vi "ZLIB Compress Directory__ogtk.vi"(6 "password (none)":string, 7 "append (create new)":T1, 8 "error in (no error)":errorcluster, 9 "include subdirectories (F)":bool, 10 "archive name (root directory with .zip ending)":path, 11 "root directory (file dialog)":path) -> (0 "error out":errorcluster, 2 "archive name out":path, 3 "root directory out":path)   [LabVIEW 2011]
doc: "This function compresses an entire directory and eventually its subdirectories into a ZIP file. The root directory must be defined and if no root directory is passed to the function it will prompt the user for such a directory with the file dialog. If no archive name is specified this function will create a file with the same name and in the same location as the root directory, by removing any possible extension from the root directory name and appending the ending .zip to it.\n\nInclude subdirectories will control if this function recursively includes any subdirectories and its content from the root directory.\n\npassword, if not empty, will encrypt all the newly added files in the archive in such a way that they can only be extracted with the password later on."
uses:
  ZLIB Open ZIP Mode__ogtk.ctl
  file/file.llb/Valid Path - Traditional__ogtk.vi
  file/file.llb/Convert File Extension (Path)__ogtk.vi
  file/file.llb/Compare Two Paths - Scalar__ogtk.vi
  ZLIB Store File__ogtk.vi
panel:
  # "Please visit http://www.OpenG.org to learn about the\nOpen Source LabVIEW software movement.\n\nNOTICE -- YOU MUST LEAVE THIS NOTICE IN PLACE.  PER THE TERMS OF THE LICENSE BELOW, YOU MAY SUBLICENSE THIS SOFTWARE \nIN ANY WAY THAT DOES NOT CONFLICT WITH THIS LICENSE.\n\n### BSD License (http://www.opensource.org/licenses/bsd-license.php) Begin ###\n \nCopyright (C) 2002-2004 Rolf Kalbermatter rolf.kalbermatter@citeng.com\nCopyright (C) 2002 Jim Kring jim@jimkring.com\n\nAll rights reserved.\n\nRedistribution and use in source and binary forms, with or without modification, are permitted provided that the following conditions are met:\n\n    * Redistributions of source code must retain the above copyright notice, this list of conditions and the following disclaimer.\n    * Redistributions in binary form must reproduce the above copyright notice, this list of conditions and the following disclaimer in the \n       documentation and/or other materials provided with the distribution.\n    * Neither the name of SciWare, James Kring, Inc., nor the names of its contributors may be used to endorse or promote products derived \n       from this software without specific prior written permission.\n\nTHIS SOFTWARE IS PROVIDED BY THE COPYRIGHT HOLDERS AND CONTRIBUTORS \"AS IS\" AND ANY EXPRESS OR IMPLIED WARRANTIES, \nINCLUDING, BUT NOT LIMITED TO, THE IMPLIED WARRANTIES OF MERCHANTABILITY AND FITNESS FOR A PARTICULAR PURPOSE ARE \nDISCLAIMED. IN NO EVENT SHALL THE COPYRIGHT OWNER OR CONTRIBUTORS BE LIABLE FOR ANY DIRECT, INDIRECT, INCIDENTAL,\n SPECIAL, EXEMPLARY, OR CONSEQUENTIAL DAMAGES (INCLUDING, BUT NOT LIMITED TO, PROCUREMENT OF SUBSTITUTE GOODS OR \nSERVICES; LOSS OF USE, DATA, OR PROFITS; OR BUSINESS INTERRUPTION) HOWEVER CAUSED AND ON ANY THEORY OF LIABILITY, \nWHETHER IN CONTRACT, STRICT LIABILITY, OR TORT (INCLUDING NEGLIGENCE OR OTHERWISE) ARISING IN ANY WAY OUT OF THE USE \nOF THIS SOFTWARE, EVEN IF ADVISED OF THE POSSIBILITY OF SUCH DAMAGE.\n\n### BSD License End ###"
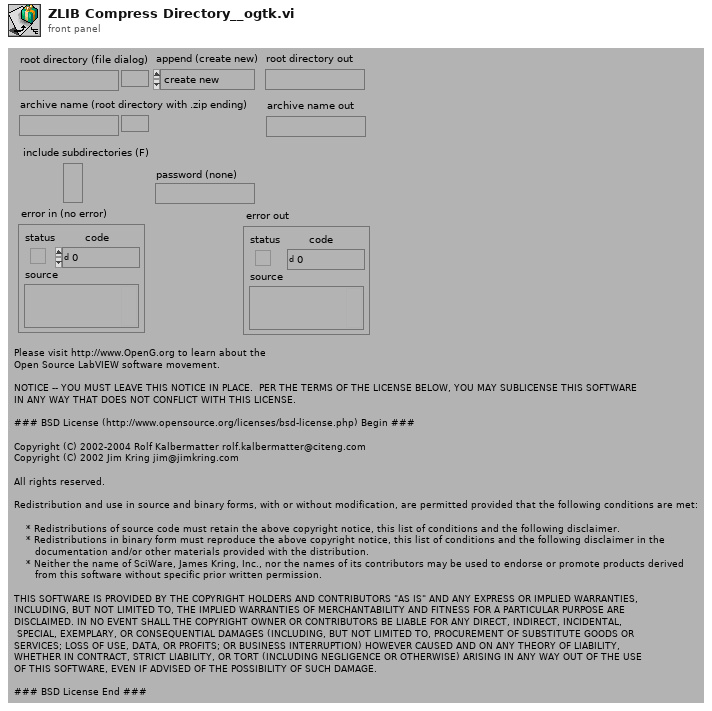
[diagram p1: front panel]
types:
  T1 = typedef "ZLIB Open ZIP Mode__ogtk.ctl" = enum16{"create new", "append to end", "append to archive"}
  T2 = enum32{"existing file", "new file", "new or existing file", "existing dir", "new dir", "new or existing dir", "existing file (use LLBs)", "new file (use LLBs)", "new or existing file (use LLBs)", "new or existing file or directory (use LLBs)", "existing dir (use LLBs)", "new dir (use LLBs)", "new or existing dir (use LLBs)", "existing file or dir", "new file or dir", "new or existing file or dir", "existing file or dir (use LLBs)", "new file or dir (use LLBs)"}
  T3 = typedef "ZLIB Zip Handle__ogtk.ctl" = refnum<k1>
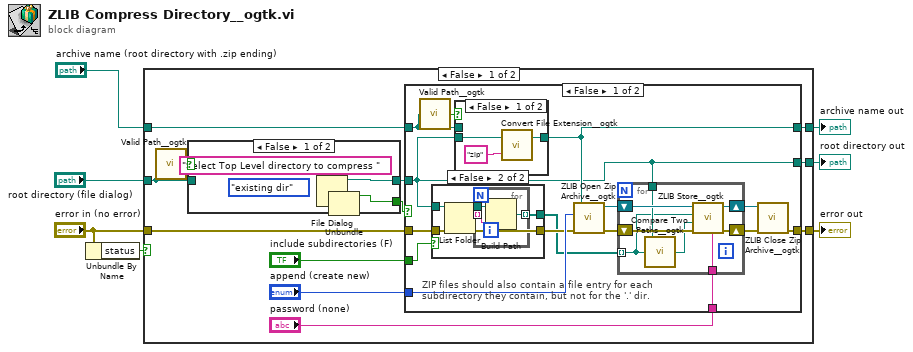
[diagram p0: block diagram]
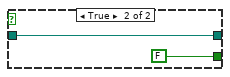
[diagram p2: hidden frame]
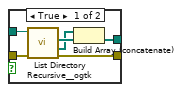
[diagram p3: hidden frame]
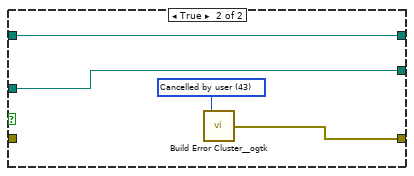
[diagram p5: hidden frame]
diagram:
  n1 = Unbundle By Name("error in (no error)") -> ("status"=w6:bool)
  n2 = case shown="False" w6 {
    tunnel: "root directory (file dialog)" -> [w16 w73]
    tunnel: "error in (no error)" -> [w13 w74]
    tunnel: [w14 w74] -> w4
    tunnel: [w12 w73] -> w3
    tunnel: [w11 w72] -> w2
    tunnel: "archive name (root directory with .zip ending)" -> [w10 w72]
    frame False {
      n3 = call-poly "Valid Path__ogtk.vi"("path"=w16) -> ("valid"=w17:bool)
      n4 = case shown="False" w17 {
        tunnel: [w22 w25] -> w19
        tunnel: [w21 FALSE ("cancelled")] -> w18
        tunnel: w16 -> [_ w25]
        frame False {
          (unwired) T2."existing dir" ("select mode (2)")
          n5 = File Dialog(7:"Select Top Level directory to compress " ("prompt")) -> (0:w20:errorcluster, 1:w21:bool, 3:w22:path)  [unwired: 6 in, 1 out]
          n6 = Unbundle(w20) -> ()  [unwired: 3 out]
        }
        frame True {
        }
      }
      n7 = case shown="False" w18 {
        tunnel: w19 -> [w31 w69]
        tunnel: w10 -> [w35 w68]
        tunnel: "include subdirectories (F)" -> [w28 _]
        tunnel: [w34 w71] -> w14
        tunnel: w13 -> [w30 _]
        tunnel: [w31 w69] -> w12
        tunnel: [w33 w68] -> w11
        tunnel: "append (create new)" -> [w32 _]
        tunnel: "password (none)" -> [w26 _]
        frame False {
          # "ZIP files should also contain a file entry for each\nsubdirectory they contain, but not for the '.' dir."
          n8 = call-poly "Valid Path__ogtk.vi"("path"=w35) -> ("valid"=w36:bool)
          n9 = case shown="False" w28 {
            tunnel: w31 -> [w46 w52]
            tunnel: [w42 w48] -> w27
            tunnel: w30 -> [w44 w51]
            tunnel: [w43 w47] -> w29
            frame True {
              n10 = call "List Directory Recursive__ogtk.vi"("error in (no error)"=w44, "Path"=w46) -> ("error out"=w43:errorcluster, "dir paths"=w41:path[], "file paths"=w45:path[])  [unwired: 6 in, 1 out]
              n11 = Build Array (concatenate)(w41, w45) -> (w42:path[])
            }
            frame False {
              n12 = List Folder(path=w52, error in=w51) -> (path out=w50:path, filenames=w49:string[], error out=w47:errorcluster)  [unwired: 2 in, 1 out]
              n13 = for {
                tunnel: w50 -> [w55]
                tunnel: w49 -> [w54] mode=indexing
                tunnel: [w53] -> w48 mode=indexing
                n14 = Build Path(base path=w55, name or relative path=w54) -> (appended path=w53:path)
              }
            }
          }
          n15 = case shown="False" w36 {
            tunnel: [w56 w59] -> w33
            tunnel: w31 -> [w57 _]
            tunnel: w35 -> [_ w59]
            frame False {
              n16 = call-poly "Convert File Extension__ogtk.vi"("new ending (none)"="zip" ("Format String"), "file name"=w57) -> ("new filename"=w56:path)  [unwired: 1 out]
            }
            frame True {
            }
          }
          n17 = call "ZLIB Open Zip Archive__ogtk.vi"("error in (no error)"=w29, "append (create new)"=w32, "archive name"=w33) -> ("error out"=w40:errorcluster, "zip Refnum"=w39:T3)  [unwired: 2 in, 1 out]
          n18 = for {
            shift-right: [w65] -> w38
            shift-left: w39 -> [w67]
            shift-right: [w64] -> w37
            shift-left: w40 -> [w66]
            tunnel: w27 -> [w62] mode=indexing
            tunnel: w31 -> [w63]
            tunnel: w26 -> [w60]
            n19 = call-poly "Compare Two Paths__ogtk.vi"("path2"=w62, "path1"=w63) -> ("relative path from 1 to 2"=w61:path)  [unwired: 1 in, 2 out]
            n20 = call-poly "ZLIB Store__ogtk.vi"("password (none)"=w60, "error in (no error)"=w66, "internal name (same as source name)"=w61, "source path"=w62, "zip Refnum"=w67) -> ("error out"=w64:errorcluster, "zip Refnum out"=w65:T3)  [unwired: 5 in]
          }
          n21 = call "ZLIB Close Zip Archive__ogtk.vi"("error in (no error)"=w37, "zip Refnum"=w38) -> ("error out"=w34:errorcluster)  [unwired: 4 in, 1 out]
        }
        frame True {
          w70 = 43 items=["No error", "Argument error", "Memory is full", "Out of zone", "End of file", "File already open", "Generic file I/O error", "File not found", "File permission error", "Disk is full", "Duplicate path", "Too many files open", "System feature not enabled", "Resource file not found", "Cannot add resource", "Resource not found", "Image not found", "Image memory error", "Pen does not exist", "Config type invalid", "Config token not found", "Config parse error", "Config memory error", "Bad external code format", "Bad external code offset", "External code not present", "Null window", "Destroy window error", "Null menu", "Print aborted", "Bad print record", "Print driver error", "Windows error during printing", "Memory error during printing", "Print dialog error", "Generic print error", "Invalid device refnum", "Device not found", "Device parameter error", "Device unit error", "Cannot open device", "Device call aborted", "Generic error", "Cancelled by user", "Object ID too low", "Object ID too high", "Object not in heap", "Unknown heap", "Unknown object (invalid DefProc)", "Unknown object (DefProc not in table)", "Message out of range", "Invalid (null) method", "Unknown message", "Manager call not supported", "Bad address", "Network operation in progress", "Network operation timed out", "Connection is busy", "Network attribute not supported", "Network error", "Address in use", "System out of memory", "Connection aborted", "Connection refused", "Not connected", "Already connected", "Connection closed", "Initialization error (interapplication manager)", "Bad occurrence", "Wait on unbound occurrence handler", "Occurrence queue overflow", "Datalog type conflict", "Unused", "Unrecognized type (interapplication manager)", "Memory corrupt", "Failed to make temporary DLL", "Old CIN version", "Drag socket not found", "Failed to load drop-object", "Failed to register OLE object", "Failed to release OLE object", "Format specifier type mismatch", "Unknown format specifier", "Too few format specifiers", "Too many format specifiers", "Scan failed", "Newer CIN version", "Error converting to variant", "Runtime menu error", "Password tampered", "Variant attribute not found", "Incompatible variant data type", "Event data is not available", "Event Store is not present", "Occurrence is not found", "Event Queue is not created", "Event info is not available", "Refnum passed is NULL", "Error retrieving Class GUID", "Error retrieving CoClass GUID", "Error retrieving TypeLib GUID.", "Bad built application magic bytes.", "Specific driver is different from the specific driver associated with the Logical Name.", "There is no session opened to the class driver.", "Max Error", "MAX - Error with config objects", "MAX - Error loading configuration", "MAX - Group not supported"]
          n22 = call "Build Error Cluster__ogtk.vi"("code"=w70) -> ("error out"=w71:errorcluster)  [unwired: 1 in]
        }
      }
    }
    frame True {
    }
  }
  "error out" <- w4
  "root directory out" <- w3
  "archive name out" <- w2
